vi "T2 Logic.vi"(7 "Upper Temperature Sensor":T1, 8 "error in (no error)":errorcluster, 11 "Data Cluster":T2={"Vesta Data Output"={"Temp_W_Raw_U"=0, "Temp_W_Raw_L"=0, "Temperature Water (F)"=0.0, "Temperature Water Compensated (F)"=0.0, "Temperature Ambient (F)"=0.0, "Setpoint Location (F)"=0.0, "Heat Request"="", "Fault Ram"="", "PWM DCDC Value"=0, "Pilot Voltage (mV)"=0.0, "Setpoint Actual (F)"=0.0, "Differential Actual (F)"=0.0, "Setpoint User (F)"=0.0, "Differential User (F)"=0.0, "Termperature FIltered -TCO (F)"=0.0, "Temp_C_Raw_1 - Sensor Voltage"="", "Temp_C_Raw_2 - Sensor Voltage"="", "Chamber Sensor Temperature (F)"=0.0, "LDO Base Temperature (F)"=0.0, "LDO Timer (sec)"=0, "Disabled (0)"=FALSE, "Warming (1)"=FALSE, "Heating (2)"=FALSE, "Cooling Data Write (3)"=FALSE, "Cooling (4)"=FALSE, "Data Read (5)"=FALSE, "N/A"=FALSE, "Temperature Trip (7)"=FALSE, "Burner"=FALSE}, "VestaTemperature"={"Water Heater Temp (°F)"=135, "Differential  (°F)"=10.0}, "Timer Application Data"={"Duty Cycle"={"Burner ON Time (Seconds)"=60.0, "Burner OFF Time (Seconds)"=60.0, "Main Burner Flag"=FALSE, "Burner Power Mode"=0}}, "Data Array"=[], "MW Output"={"TC1-Channel 021"=0.0, "TC2-Channel 022"=0.0, "TC3-Channel 023"=0.0, "TC4-Channel 024"=0.0, "TC5-Channel 025"=0.0, "TC6-Channel 026"=0.0, "TC7-Channel 017"=0.0, "TC8-Channel 028"=0.0, "TC9-Channel 029"=0.0, "TC10-Channel 030"=0.0, "TC Tree Average"=0.0, "TC DWN- Channel 027"=0.0, "RTDin-Channel 031"=0.0, "RTDout-Channel 032"=0.0, "RTDamb-Channel 033"=0.0, "PSI1-Channel 011"=0.0, "PSI2-Channel 012"=0.0, "PSI3-Channel 013"=0.0, "PSI4-Channel 014"=0.0, "UE State-Channel 015"=0.0, "LE State-Channel 016"=0.0, "Module 4 Relay Status Output"={"INTELLIFAUCET TEMP(T)/FLOW(F) (CH 041)"=FALSE, "INTELLIFAUCET READY (CH 042)"=FALSE, "INTELLIFAUCET START (CH 043)"=FALSE, "INTELLIFAUCET STOP (CH 044)"=FALSE, "MAIN POWER RELAY (CH 047)"=FALSE, "NOT USED (CH 045)"=FALSE, "NOT USED (CH 046)"=FALSE, "PURGE VALVE RELAY (CH 048)"=FALSE, "OUTLET VALVE RELAY (CH 049)"=FALSE, "INLET VALVE RELAY (CH 050)"=FALSE, "Intellifaucet (% Open)"=0.0, "Proportioning Valve (%Open)"=0.0, "Intellifaucet Temp Setpoint (F)"=0.0}}} {"VestaTemperature"."Water Heater Temp (°F)" min=32 max=203}) -> (0 "error out":errorcluster, 3 "Data Cluster Output":T2={"Vesta Data Output"={"Temp_W_Raw_U"=0, "Temp_W_Raw_L"=0, "Temperature Water (F)"=0.0, "Temperature Water Compensated (F)"=0.0, "Temperature Ambient (F)"=0.0, "Setpoint Location (F)"=0.0, "Heat Request"="", "Fault Ram"="", "PWM DCDC Value"=0, "Pilot Voltage (mV)"=0.0, "Setpoint Actual (F)"=0.0, "Differential Actual (F)"=0.0, "Setpoint User (F)"=0.0, "Differential User (F)"=0.0, "Termperature FIltered -TCO (F)"=0.0, "Temp_C_Raw_1 - Sensor Voltage"="", "Temp_C_Raw_2 - Sensor Voltage"="", "Chamber Sensor Temperature (F)"=0.0, "LDO Base Temperature (F)"=0.0, "LDO Timer (sec)"=0, "Disabled (0)"=FALSE, "Warming (1)"=FALSE, "Heating (2)"=FALSE, "Cooling Data Write (3)"=FALSE, "Cooling (4)"=FALSE, "Data Read (5)"=FALSE, "N/A"=FALSE, "Temperature Trip (7)"=FALSE, "Burner"=FALSE}, "VestaTemperature"={"Water Heater Temp (°F)"=135, "Differential  (°F)"=10.0}, "Timer Application Data"={"Duty Cycle"={"Burner ON Time (Seconds)"=60.0, "Burner OFF Time (Seconds)"=60.0, "Main Burner Flag"=FALSE, "Burner Power Mode"=0}}, "Data Array"=[], "MW Output"={"TC1-Channel 021"=0.0, "TC2-Channel 022"=0.0, "TC3-Channel 023"=0.0, "TC4-Channel 024"=0.0, "TC5-Channel 025"=0.0, "TC6-Channel 026"=0.0, "TC7-Channel 017"=0.0, "TC8-Channel 028"=0.0, "TC9-Channel 029"=0.0, "TC10-Channel 030"=0.0, "TC Tree Average"=0.0, "TC DWN- Channel 027"=0.0, "RTDin-Channel 031"=0.0, "RTDout-Channel 032"=0.0, "RTDamb-Channel 033"=0.0, "PSI1-Channel 011"=0.0, "PSI2-Channel 012"=0.0, "PSI3-Channel 013"=0.0, "PSI4-Channel 014"=0.0, "UE State-Channel 015"=0.0, "LE State-Channel 016"=0.0, "Module 4 Relay Status Output"={"INTELLIFAUCET TEMP(T)/FLOW(F) (CH 041)"=FALSE, "INTELLIFAUCET READY (CH 042)"=FALSE, "INTELLIFAUCET START (CH 043)"=FALSE, "INTELLIFAUCET STOP (CH 044)"=FALSE, "MAIN POWER RELAY (CH 047)"=FALSE, "NOT USED (CH 045)"=FALSE, "NOT USED (CH 046)"=FALSE, "PURGE VALVE RELAY (CH 048)"=FALSE, "OUTLET VALVE RELAY (CH 049)"=FALSE, "INLET VALVE RELAY (CH 050)"=FALSE, "Intellifaucet (% Open)"=0.0, "Proportioning Valve (%Open)"=0.0, "Intellifaucet Temp Setpoint (F)"=0.0}}} {"VestaTemperature"."Water Heater Temp (°F)" min=32 max=203}, 4 "Send_Vesta_Message":i32, 6 "Send_Timer_Message":i32)   [LabVIEW 2023]
uses:
  controls/UI Data.ctl
  Drivers/Resideo Gas Valve/Type Definitions/Vesta Info.ctl
  Drivers/Resideo Gas Valve/Type Definitions/Temperature Control.ctl
  controls/Timer Application Cluster.ctl
  controls/Burner Duty Cycle.ctl
  Hybrid Water Heater/Type Definitions/HEWH MW100 Data Cluster.ctl
  Hybrid Water Heater/Custom Instrument Control/MW100/Type Definitions/HEWH Module 4 Relay Status.ctl
  controls/Upper Temperature Sensor.ctl
  <vilib>/Utility/error.llb/whitespace.ctl
  <vilib>/Utility/error.llb/Trim Whitespace One-Sided.vi
panel:
  out "upper_is_high":i32
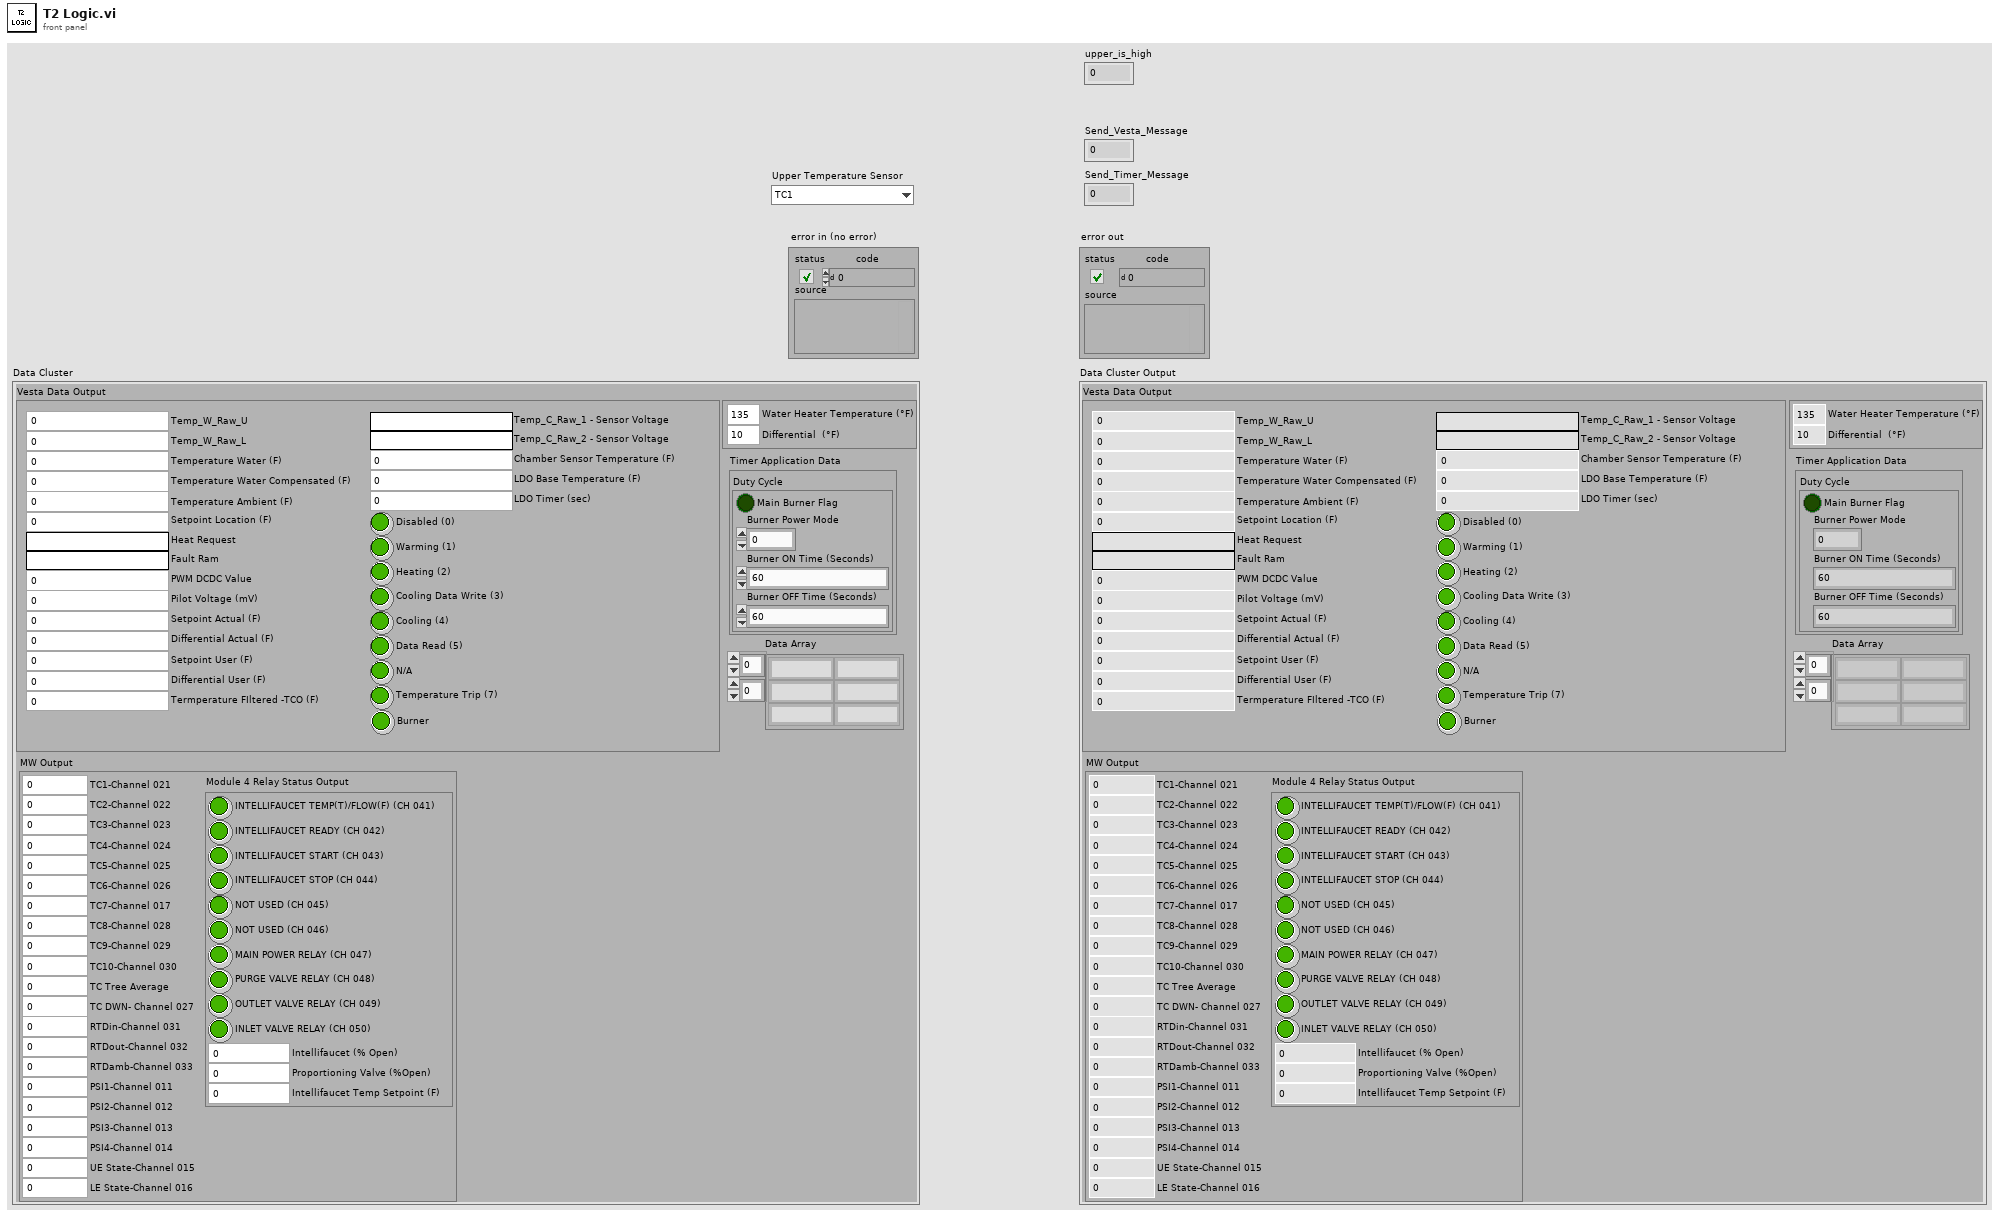
[diagram p1: front panel]
types:
  T1 = typedef "Upper Temperature Sensor.ctl" = enum16{"TC1", "TC2", "TC3", "TC4", "TC5", "TC6"}
  T2 = typedef "UI Data.ctl" = cluster{"Vesta Data Output":T3, "VestaTemperature":T4, "Timer Application Data":T5, "Data Array":string[][], "MW Output":T7}
  T3 = typedef "Vesta Info.ctl" = cluster{"Temp_W_Raw_U":u16, "Temp_W_Raw_L":u16, "Temperature Water (F)":dbl, "Temperature Water Compensated (F)":dbl, "Temperature Ambient (F)":dbl, "Setpoint Location (F)":dbl, "Heat Request":string, "Fault Ram":string, "PWM DCDC Value":u16, "Pilot Voltage (mV)":dbl, "Setpoint Actual (F)":dbl, "Differential Actual (F)":dbl, "Setpoint User (F)":dbl, "Differential User (F)":dbl, "Termperature FIltered -TCO (F)":dbl, "Temp_C_Raw_1 - Sensor Voltage":string, "Temp_C_Raw_2 - Sensor Voltage":string, "Chamber Sensor Temperature (F)":dbl, "LDO Base Temperature (F)":dbl, "LDO Timer (sec)":i16, "Disabled (0)":bool, "Warming (1)":bool, "Heating (2)":bool, "Cooling Data Write (3)":bool, "Cooling (4)":bool, "Data Read (5)":bool, "N/A":bool, "Temperature Trip (7)":bool, "Burner":bool}
  T4 = typedef "Temperature Control.ctl" = cluster{"Water Heater Temp (°F)":u16, "Differential  (°F)":dbl}
  T5 = typedef "Timer Application Cluster.ctl" = cluster{"Duty Cycle":T6}
  T6 = typedef "Burner Duty Cycle.ctl" = cluster{"Burner ON Time (Seconds)":dbl, "Burner OFF Time (Seconds)":dbl, "Main Burner Flag":bool, "Burner Power Mode":u8}
  T7 = typedef "HEWH MW100 Data Cluster.ctl" = cluster{"TC1-Channel 021":dbl, "TC2-Channel 022":dbl, "TC3-Channel 023":dbl, "TC4-Channel 024":dbl, "TC5-Channel 025":dbl, "TC6-Channel 026":dbl, "TC7-Channel 017":dbl, "TC8-Channel 028":dbl, "TC9-Channel 029":dbl, "TC10-Channel 030":dbl, "TC Tree Average":dbl, "TC DWN- Channel 027":dbl, "RTDin-Channel 031":dbl, "RTDout-Channel 032":dbl, "RTDamb-Channel 033":dbl, "PSI1-Channel 011":dbl, "PSI2-Channel 012":dbl, "PSI3-Channel 013":dbl, "PSI4-Channel 014":dbl, "UE State-Channel 015":dbl, "LE State-Channel 016":dbl, "Module 4 Relay Status Output":T8}
  T8 = typedef "HEWH Module 4 Relay Status.ctl" = cluster{"INTELLIFAUCET TEMP(T)/FLOW(F) (CH 041)":bool, "INTELLIFAUCET READY (CH 042)":bool, "INTELLIFAUCET START (CH 043)":bool, "INTELLIFAUCET STOP (CH 044)":bool, "MAIN POWER RELAY (CH 047)":bool, "NOT USED (CH 045)":bool, "NOT USED (CH 046)":bool, "PURGE VALVE RELAY (CH 048)":bool, "OUTLET VALVE RELAY (CH 049)":bool, "INLET VALVE RELAY (CH 050)":bool, "Intellifaucet (% Open)":dbl, "Proportioning Valve (%Open)":dbl, "Intellifaucet Temp Setpoint (F)":dbl}
  T9 = typedef "whitespace.ctl" = u16
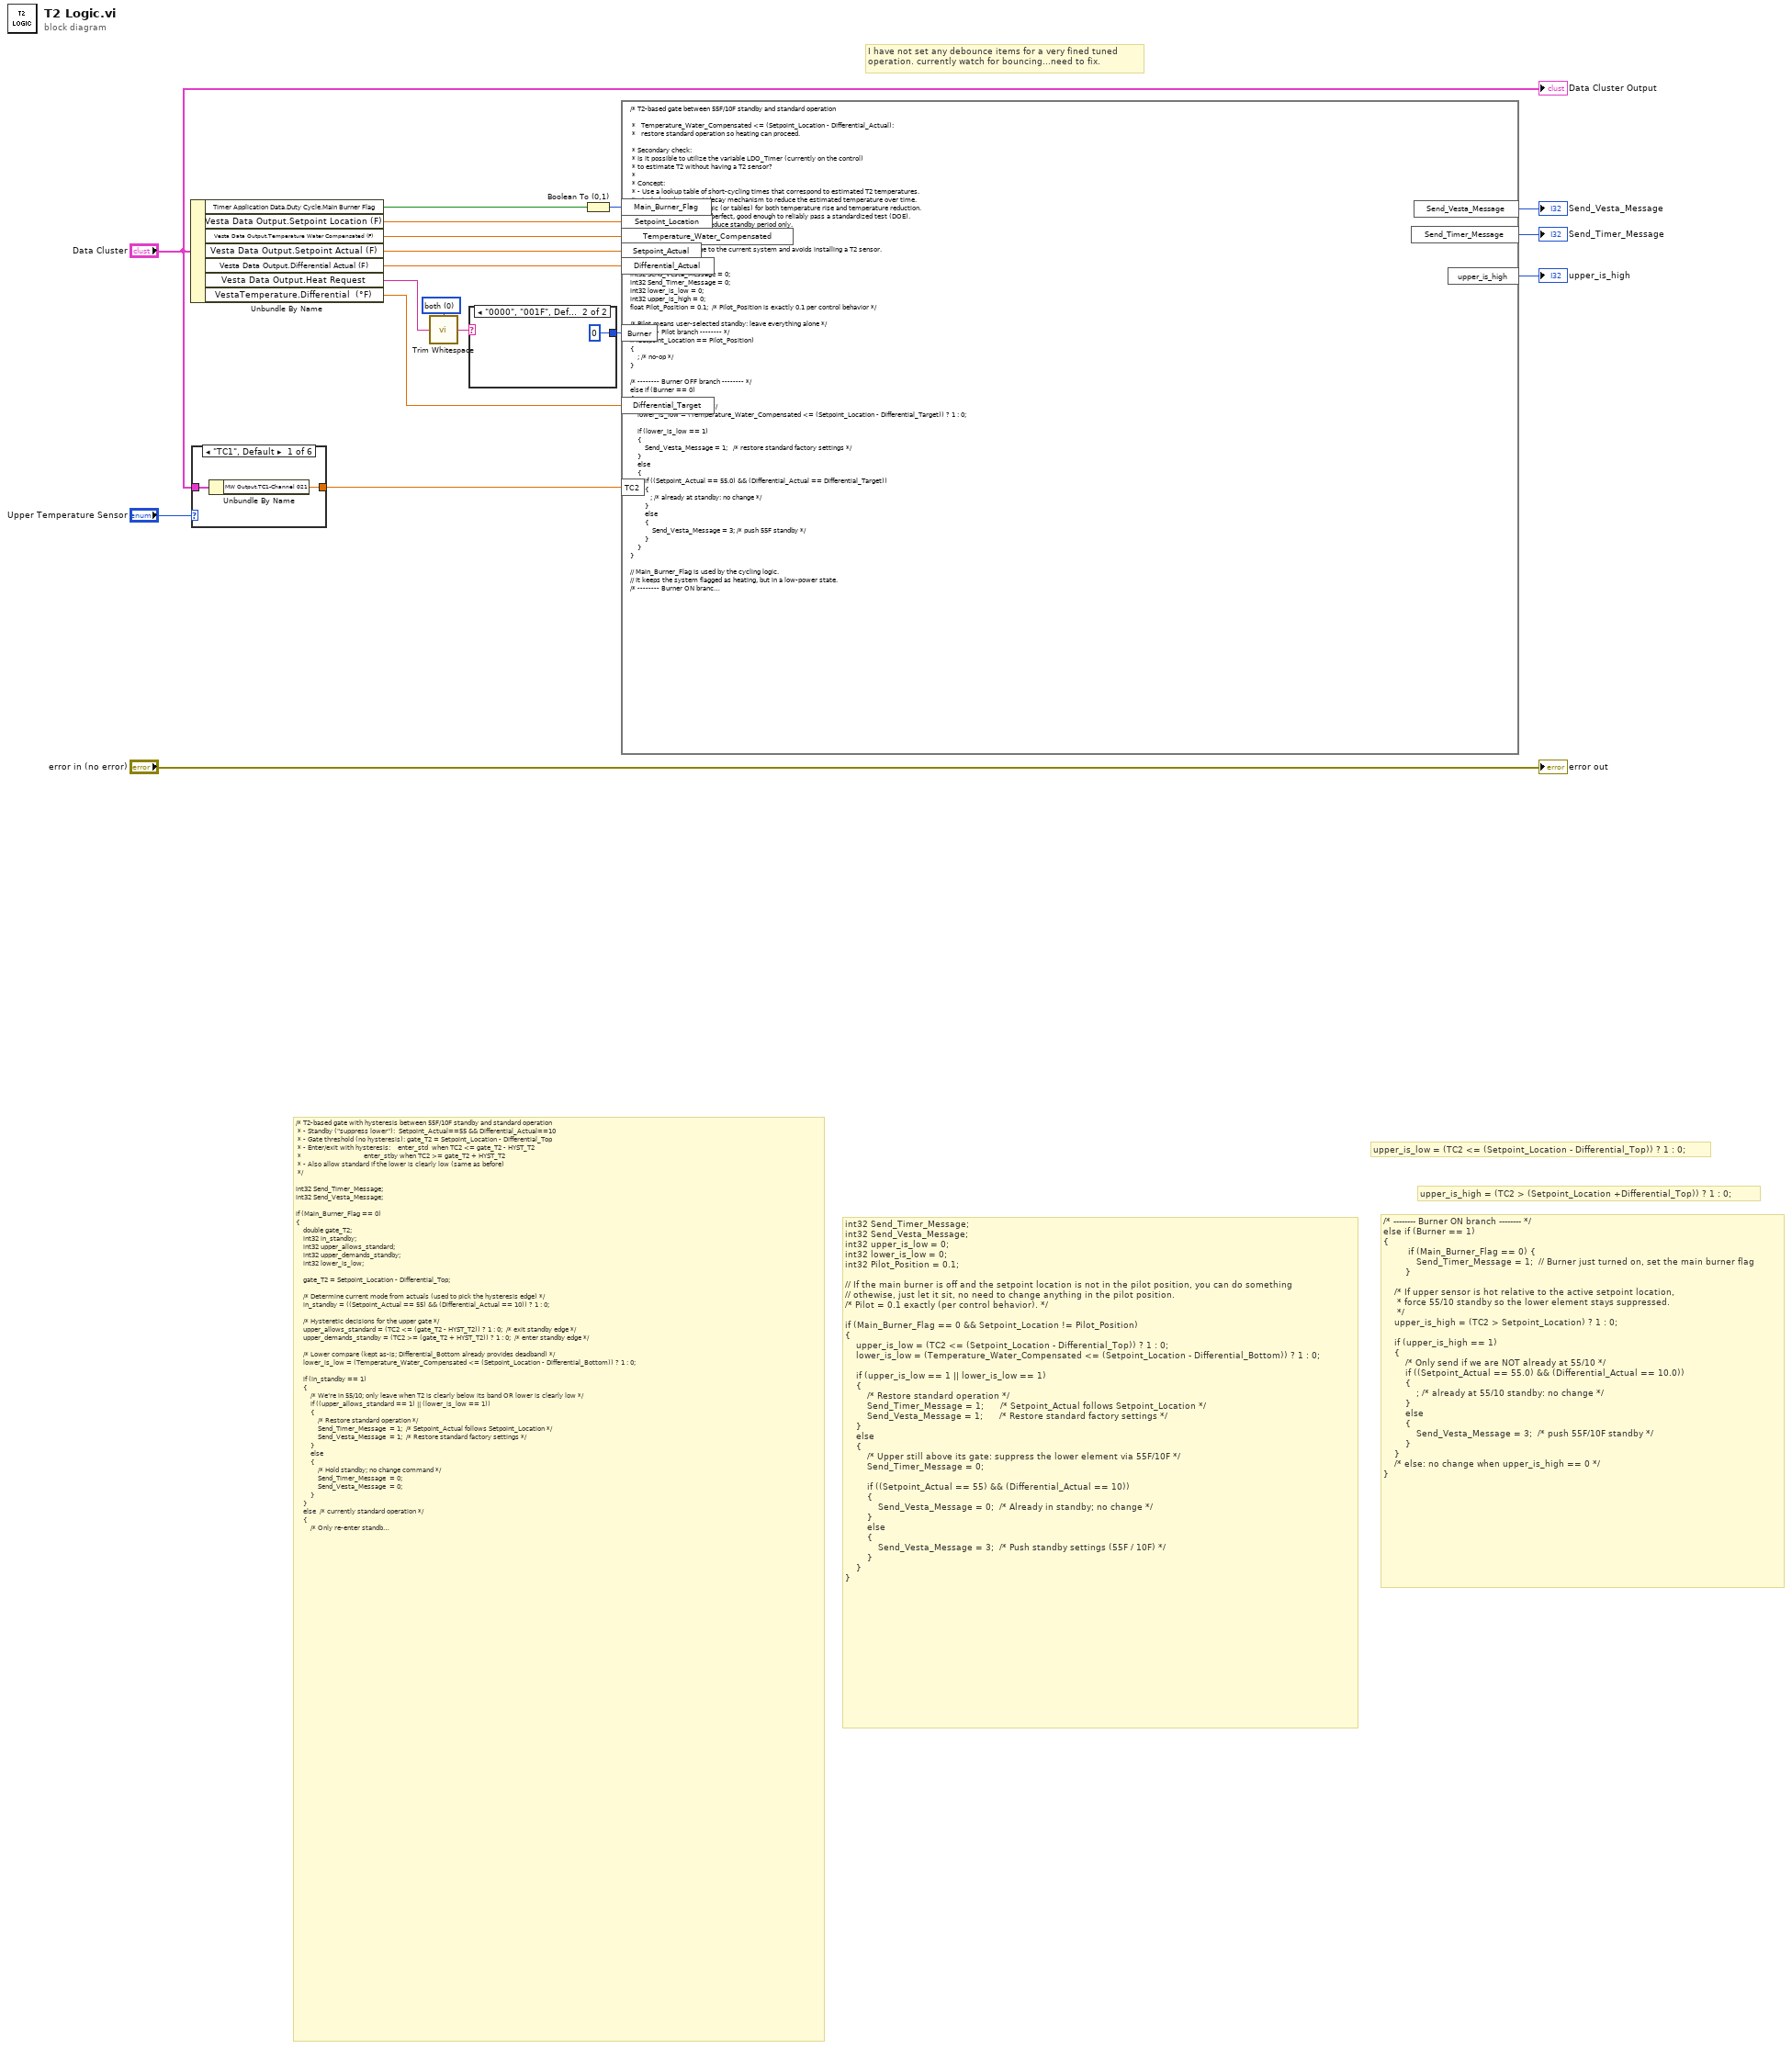
[diagram p0: block diagram]
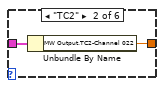
[diagram p2: hidden frame]
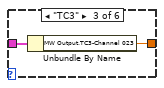
[diagram p3: hidden frame]
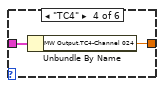
[diagram p4: hidden frame]
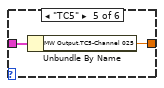
[diagram p5: hidden frame]
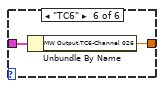
[diagram p6: hidden frame]
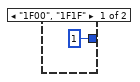
[diagram p7: hidden frame]
diagram:
  w9 = T9 0 items=["both", "start of string", "end of string"] ("location (both)")
  # "I have not set any debounce items for a very fined tuned \noperation. currently watch for bouncing...need to fix."
  # "/* -------- Burner ON branch -------- */\nelse if (Burner == 1)\n{\n         if (Main_Burner_Flag == 0) {\n            Send_Timer_Message = 1;  // Burner just turned on, set the main burner flag\n        }\n\n    /* If upper sensor is hot relative to the active setpoint location,\n     * force 55/10 standby so the lower element stays suppressed.\n     */\n    upper_is_high = (TC2 > Setpoint_Location) ? 1 : 0;\n\n    if (upper_is_high == 1)\n    {\n        /* Only send if we are NOT already at 55/10 */\n        if ((Setpoint_Actual == 55.0) && (Differential_Actual == 10.0))\n        {\n            ; /* already at 55/10 standby: no change */\n        }\n        else\n        {\n            Send_Vesta_Message = 3;  /* push 55F/10F standby */\n        }\n    }\n    /* else: no change when upper_is_high == 0 */\n}"
  # "upper_is_high = (TC2 > (Setpoint_Location +Differential_Top)) ? 1 : 0;"
  # "upper_is_low = (TC2 <= (Setpoint_Location - Differential_Top)) ? 1 : 0;"
  # "int32 Send_Timer_Message;\nint32 Send_Vesta_Message;\nint32 upper_is_low = 0;\nint32 lower_is_low = 0;\nint32 Pilot_Position = 0.1;\n\n// If the main burner is off and the setpoint location is not in the pilot position, you can do something\n// othewise, just let it sit, no need to change anything in the pilot position.\n/* Pilot = 0.1 exactly (per control behavior). */\n\nif (Main_Burner_Flag == 0 && Setpoint_Location != Pilot_Position)\n{\n    upper_is_low = (TC2 <= (Setpoint_Location - Differential_Top)) ? 1 : 0;\n    lower_is_low = (Temperature_Water_Compensated <= (Setpoint_Location - Differential_Bottom)) ? 1 : 0;\n\n    if (upper_is_low == 1 || lower_is_low == 1)\n    {\n        /* Restore standard operation */\n        Send_Timer_Message = 1;      /* Setpoint_Actual follows Setpoint_Location */\n        Send_Vesta_Message = 1;      /* Restore standard factory settings */\n    }\n    else\n    {\n        /* Upper still above its gate: suppress the lower element via 55F/10F */\n        Send_Timer_Message = 0;\n\n        if ((Setpoint_Actual == 55) && (Differential_Actual == 10))\n        {\n            Send_Vesta_Message = 0;  /* Already in standby; no change */\n        }\n        else\n        {\n            Send_Vesta_Message = 3;  /* Push standby settings (55F / 10F) */\n        }\n    }\n}"
  # "/* T2-based gate with hysteresis between 55F/10F standby and standard operation\n * - Standby (\"suppress lower\"):  Setpoint_Actual==55 && Differential_Actual==10\n * - Gate threshold (no hysteresis): gate_T2 = Setpoint_Location - Differential_Top\n * - Enter/exit with hysteresis:    enter_std  when TC2 <= gate_T2 - HYST_T2\n *                                  enter_stby when TC2 >= gate_T2 + HYST_T2\n * - Also allow standard if the lower is clearly low (same as before)\n */\n\nint32 Send_Timer_Message;\nint32 Send_Vesta_Message;\n\nif (Main_Burner_Flag == 0)\n{\n    double gate_T2;\n    int32 in_standby;\n    int32 upper_allows_standard;\n    int32 upper_demands_standby;\n    int32 lower_is_low;\n\n    gate_T2 = Setpoint_Location - Differential_Top;\n\n    /* Determine current mode from actuals (used to pick the hysteresis edge) */\n    in_standby = ((Setpoint_Actual == 55) && (Differential_Actual == 10)) ? 1 : 0;\n\n    /* Hysteretic decisions for the upper gate */\n    upper_allows_standard = (TC2 <= (gate_T2 - HYST_T2)) ? 1 : 0;  /* exit standby edge */\n    upper_demands_standby = (TC2 >= (gate_T2 + HYST_T2)) ? 1 : 0;  /* enter standby edge */\n\n    /* Lower compare (kept as-is; Differential_Bottom already provides deadband) */\n    lower_is_low = (Temperature_Water_Compensated <= (Setpoint_Location - Differential_Bottom)) ? 1 : 0;\n\n    if (in_standby == 1)\n    {\n        /* We’re in 55/10; only leave when T2 is clearly below its band OR lower is clearly low */\n        if ((upper_allows_standard == 1) || (lower_is_low == 1))\n        {\n            /* Restore standard operation */\n            Send_Timer_Message  = 1;  /* Setpoint_Actual follows Setpoint_Location */\n            Send_Vesta_Message  = 1;  /* Restore standard factory settings */\n        }\n        else\n        {\n            /* Hold standby; no change command */\n            Send_Timer_Message  = 0;\n            Send_Vesta_Message  = 0;\n        }\n    }\n    else  /* currently standard operation */\n    {\n        /* Only re-enter standby when T2 is clearly above its band */\n        if (upper_demands_standby == 1)\n        {\n            Send_Timer_Message = 0;   /* go to standby path */\n            if ((Setpoint_Actual == 55) && (Differential_Actual == 10))\n                Send_Vesta_Message = 0;  /* already standby */\n            else\n                Send_Vesta_Message = 3;  /* push 55F / 10F */\n        }\n        else\n        {\n            /* Stay standard; do nothing */\n            Send_Timer_Message  = 0;\n            Send_Vesta_Message  = 0;\n        }\n    }\n}"
  n1 = Unbundle By Name("Data Cluster") -> ("Timer Application Data.Duty Cycle.Main Burner Flag"=w12:bool, "Vesta Data Output.Setpoint Location (F)"=w17:dbl, "Vesta Data Output.Temperature Water Compensated (F)"=w16:dbl, "Vesta Data Output.Setpoint Actual (F)"=w15:dbl, "Vesta Data Output.Differential Actual (F)"=w14:dbl, "Vesta Data Output.Heat Request"=w7:string, "VestaTemperature.Differential  (°F)"=w4:dbl)
  n2 = case shown="\"TC1\", Default" "Upper Temperature Sensor" {
    tunnel: "Data Cluster" -> [w20 w22 w24 w26 w28 w30]
    tunnel: [w19 w21 w23 w25 w27 w29] -> w2
    frame "TC1", Default {
      n3 = Unbundle By Name(w20) -> ("MW Output.TC1-Channel 021"=w19:dbl)
    }
    frame "TC2" {
      n4 = Unbundle By Name(w22) -> ("MW Output.TC2-Channel 022"=w21:dbl)
    }
    frame "TC3" {
      n5 = Unbundle By Name(w24) -> ("MW Output.TC3-Channel 023"=w23:dbl)
    }
    frame "TC4" {
      n6 = Unbundle By Name(w26) -> ("MW Output.TC4-Channel 024"=w25:dbl)
    }
    frame "TC5" {
      n7 = Unbundle By Name(w28) -> ("MW Output.TC5-Channel 025"=w27:dbl)
    }
    frame "TC6" {
      n8 = Unbundle By Name(w30) -> ("MW Output.TC6-Channel 026"=w29:dbl)
    }
  }
  n9 = call <vilib>:"Trim Whitespace.vi"("string"=w7, "location (both)"=w9) -> ("trimmed string"=w8:string)
  n10 = case shown="\"0000\", \"001F\", Default" w8 {
    tunnel: [1 0] -> w6
    frame "1F00", "1F1F" {
    }
    frame "0000", "001F", Default {
    }
  }
  n11 = Boolean To (0,1)(Boolean=w12) -> (0, 1=w11:i16)
  n12 = formula code="/* T2-based gate between 55F/10F standby and standard operation\n\n *   Temperature_Water_Compensated <= (Setpoint_Location - Differential_Actual):\n *   restore standard operation so heating can proceed.\n\n * Secondary check:\n * Is it possible to utilize the variable LDO_Timer (currently on the control)\n * to estimate T2 without having a T2 sensor?\n *\n * Concept:\n * - Use a lookup table of short-cycling times that correspond to estimated T2 temperatures.\n * - Include a decrement/decay mechanism to reduce the estimated temperature over time.\n * - This implies having logic (or tables) for both temperature rise and temperature reduction.\n * - It does not have to be perfect, good enough to reliably pass a standardized test (DOE). \n * - Might try to cycle to reduce standby period only. \n *\n * Benefit:\n * - Prevents any change to the current system and avoids installing a T2 sensor.\n\n/* defaults: */\nint32 Send_Vesta_Message = 0;\nint32 Send_Timer_Message = 0;\nint32 lower_is_low = 0;\nint32 upper_is_high = 0;\nfloat Pilot_Position = 0.1;  /* Pilot_Position is exactly 0.1 per control behavior */\n\n/* Pilot means user-selected standby: leave everything alone */\n/* -------- Pilot branch -------- */\nif (Setpoint_Location == Pilot_Position)\n{\n    ; /* no-op */\n}\n\n/* -------- Burner OFF branch -------- */\nelse if (Burner == 0)\n{\n    /* T1-Differential Check */\n    lower_is_low = (Temperature_Water_Compensated <= (Setpoint_Location - Differential_Target)) ? 1 : 0;\n\n    if (lower_is_low == 1)\n    {\n        Send_Vesta_Message = 1;   /* restore standard factory settings */\n    }\n    else\n    {\n        if ((Setpoint_Actual == 55.0) && (Differential_Actual == Differential_Target))\n        {\n           ; /* already at standby: no change */\n        }\n        else\n        {\n            Send_Vesta_Message = 3; /* push 55F standby */\n        }\n    }\n}\n\n// Main_Burner_Flag is used by the cycling logic.\n// It keeps the system flagged as heating, but in a low-power state.\n/* -------- Burner ON branch -------- */\nelse if (Burner == 1)\n{\n    /* 0) Edge detect: burner just turned ON */\n    if (Main_Burner_Flag == 0) {\n        Send_Timer_Message = 1;    // burner-on edge\n        // Get Temperature snap shots here. TC_Bottom and TC_Top\n        // Clear any Large_Draw_Lockout\n    }\n\n    /* 1) If upper sensor is high vs. active setpoint,\n          force 55f standby so the lower element stays suppressed. */\n    upper_is_high = (TC2 > Setpoint_Location) ? 1 : 0;\n\n    if (upper_is_high == 1)\n    {\n        /* Only send if we are NOT already at 55f */\n        if (!(Setpoint_Actual == 55.0 && Differential_Actual == Differential_Target))\n        {\n            Send_Vesta_Message = 3;    /* push standby */\n        }\n        /* else: already at standby — no change */\n    }\n    /* else: upper_is_high == 0 — no change */\n}"("Burner"=w6, "Setpoint_Location"=w17, "Temperature_Water_Compensated"=w16, "Setpoint_Actual"=w15, "Differential_Actual"=w14, "TC2"=w2, "Main_Burner_Flag"=w11, "Differential_Target"=w4) -> ("Send_Vesta_Message"=→"Send_Vesta_Message":i32, "upper_is_high"=→"upper_is_high":i32, "Send_Timer_Message"=→"Send_Timer_Message":i32)
  "Data Cluster Output" <- "Data Cluster"
  "error out" <- "error in (no error)"
